vi "test.vi"() -> ()   [LabVIEW 2011]
panel:
  in  "stop":bool
  out "SC":bool
  out "S5":bool
  out "S4":bool
  out "S3":bool
  out "S2":bool
  out "S1":bool
  out "really lost":bool
  out "line found":bool
  out "error":dbl
  in  "last error":dbl=15000.0 min=10240.0 max=19650.0 step=100.0
  in  "S5in":u16=15000 min=10240 max=19650 step=100
  in  "S4in":u16=15000 min=10240 max=19650 step=100
  in  "S3in":u16=15000 min=10240 max=19650 step=100
  in  "S2in":u16=15000 min=10240 max=19650 step=100
  in  "S1in":u16=15000 min=10240 max=19650 step=100
  in  "SCin":u16=15000 min=10240 max=19650 step=100
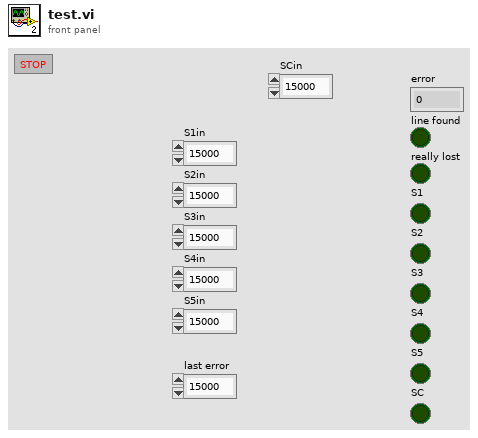
[diagram p1: front panel]
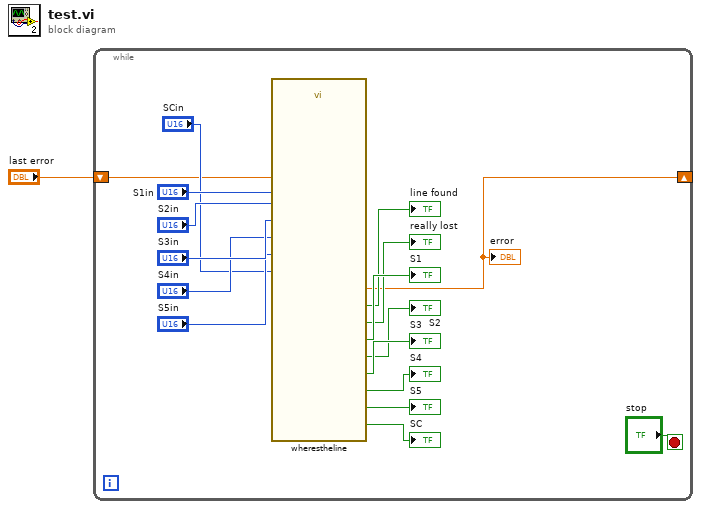
[diagram p0: block diagram]
diagram:
  n1 = while {
    shift-right: [w2] -> _
    shift-left: "last error" -> [w11]
    stop <- "stop" stop-if-true
    n2 = call "wherestheline.vi"("SCin"="SCin", "S1in"="S1in", "S2in"="S2in", "S3in"="S3in", "S4in"="S4in", "S5in"="S5in", "last error"=w11) -> ("SC"=→"SC":bool, "error"=w2:dbl, "line found"=→"line found":bool, "really lost"=→"really lost":bool, "S1"=→"S1":bool, "S2"=→"S2":bool, "S3"=→"S3":bool, "S4"=→"S4":bool, "S5"=→"S5":bool)  [unwired: 12 in]
    "error" <- w2
  }
